vi "CUST Read Next Frame.vi"(10 "pseudoPdcId":i32, 11 "timeoutMs":i32) -> (0 "function return":i32)   [LabVIEW 2013, in "C37118-DLL.lvlib"]
doc: "STRONGRIDIEEEC37118DLL_API int __cdecl readNextFrame( int32_t timeoutMs, int32_t pseudoPdcId);"
uses:
  C37118-DLL.lvlib
  builds/StrongridDLL/StrongridDLL.dll
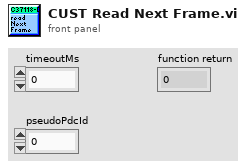
[diagram p1: front panel]
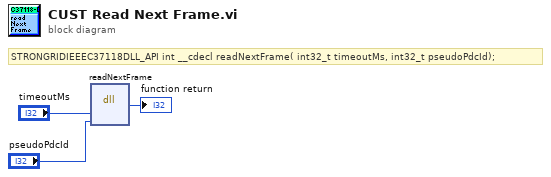
[diagram p0: block diagram]
diagram:
  # "STRONGRIDIEEEC37118DLL_API int __cdecl readNextFrame( int32_t timeoutMs, int32_t pseudoPdcId);"
  n1 = dll-call lib="C:/dev/OSS/S3DK/builds/StrongridDLL/StrongridDLL.*" fn="readNextFrame"("timeoutMs"="timeoutMs", "pseudoPdcId"="pseudoPdcId") -> (→"function return":i32)  [unwired: 5 in, 2 out]
